vi "LVClass_WavefrontCorrectorSet Get Parameter Type.vi"(0 "WavefrontCorrectorSet in":refnum<class "WavefrontCorrectorSet.lvclass">, 5 "parameter_name":string, 11 "error in (no error)":errorcluster) -> (4 "WavefrontCorrectorSet out":refnum<class "WavefrontCorrectorSet.lvclass">, 6 "Type":T1, 15 "error out":errorcluster)   [LabVIEW 2020, in "WavefrontCorrectorSet.lvclass"]
doc: "WavefrontCorrector parameter type getter given its name which should have been\nread with Imop_WavefrontCorrectorSet_GetParameterName.\n\n--------------------------------------------------------------------------------\n\n<B>wavefrontcorrector_setIn </B> : WavefrontCorrectorSet object.\n<B>wavefrontcorrector_setOut </B> : WavefrontCorrectorSet object.\n<B>parameter_name </B> : Parameter name.\n<B>type </B> : Parameter type.\n<B>ErrorIn </B> : Error\n<B>ErrorOut </B> : Error\n\n--------------------------------------------------------------------------------"
uses:
  WavefrontCorrectorSet.lvclass
  Controls/CameraParameters_Type.ctl
  WavefrontCorrectorSet.lvclass/WavefrontCorrectorSet.ctl
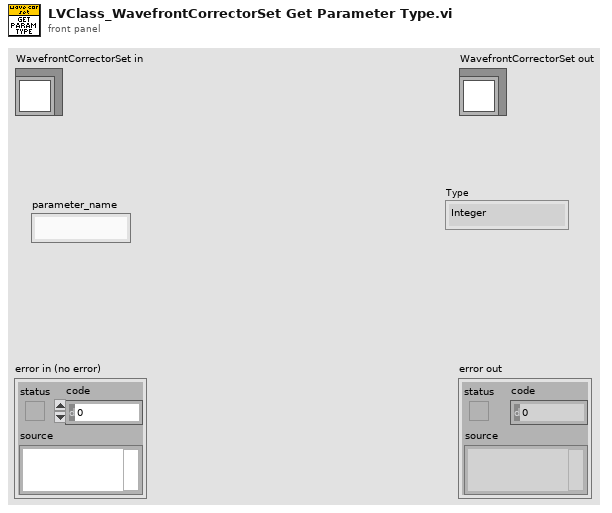
[diagram p1: front panel]
types:
  T1 = typedef "CameraParameters_Type.ctl" = enum16{"Integer", "Real", "String", "Boolean"}
  T2 = typedef "ClassID.ctl" = i64
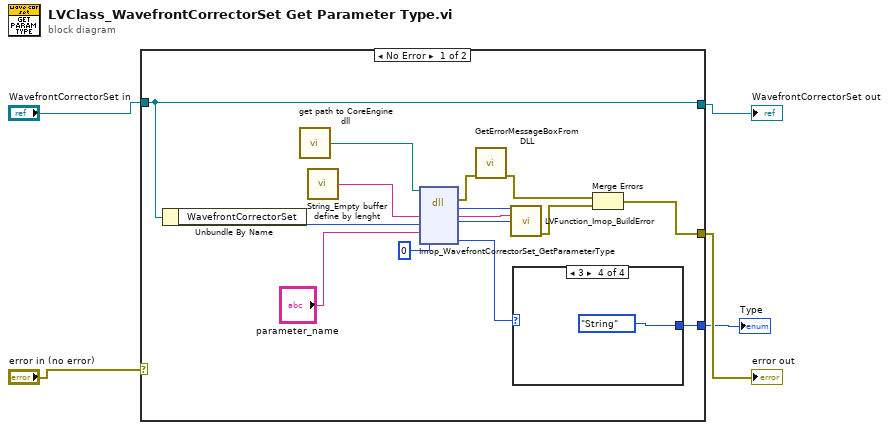
[diagram p0: block diagram]
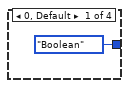
[diagram p2: hidden frame]
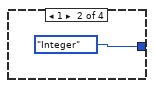
[diagram p3: hidden frame]
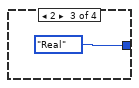
[diagram p4: hidden frame]
diagram:
  n1 = case shown="No Error" "error in (no error)" {
    selector: "error in (no error)" -> [_ w25]
    tunnel: "WavefrontCorrectorSet in" -> [w7 w26]
    tunnel: [w7 w26] -> w3
    tunnel: [w8 w25] -> w2
    tunnel: [w12 _] -> w1
    frame No Error {
      n2 = Unbundle By Name(w7) -> ("WavefrontCorrectorSet"=w11:T2)
      n3 = call "get path to CoreEngine dll.vi"() -> ("path to wavekit library"=w15:path)  [unwired: 14 in, 1 out]
      n4 = call "String_Empty buffer define by lenght.vi"() -> ("Empty buffer"=w18:string)  [unwired: 1 in]
      n5 = dll-call lib="D:/soft/HASO_v3/C_interface/Sources/Build/vc100/Release/c_interface_vc100.dll" fn="Imop_WavefrontCorrectorSet_GetParameterType"(path in=w15, "message"=w18, "objet"=w11, "parameter_name"="parameter_name", "type"=u32 0) -> (error out=w14:errorcluster, "return type"=w20:i32, "message"=w19:string, "objet"=w6:i64, "type"=w13:i32)  [unwired: 3 in, 1 out]
      n6 = call "GetErrorMessageBoxFromDLL.vi"("error IN"=w14) -> ("error OUT"=w10:errorcluster)  [unwired: 10 in]
      n7 = call "LVFunction_Imop_BuildError.vi"("code"=w20, "String to Prepend to source (\"\")"=w19, "Adresse"=w6) -> ("error out"=w9:errorcluster)  [unwired: 12 in]
      n8 = case shown="3" w13 {
        tunnel: [CameraParameters_Type."Boolean" ("Type 2") CameraParameters_Type."Integer" ("Type 2") CameraParameters_Type."Real" ("Type 2") CameraParameters_Type."String" ("Type 2")] -> w12
        frame 0, Default {
        }
        frame 1 {
        }
        frame 2 {
        }
        frame 3 {
        }
      }
      n9 = Merge Errors(w10, w9) -> (w8:errorcluster)
    }
    frame Error {
    }
  }
  "error out" <- w2
  "WavefrontCorrectorSet out" <- w3
  "Type" <- w1
